vi "Update post-assembly comments.vi"(8 "error in (no error)":errorcluster, 10 "Tray N Pos M":T1, 11 "Stack in":refnum<class "Stack.lvclass">) -> (0 "error out":errorcluster, 3 "Stack out":refnum<class "Stack.lvclass">)   [LabVIEW 2021, in "Stack.lvclass"]
uses:
  Stack.lvclass
  Stack.lvclass/Stack.ctl
panel:
  # "This is only to be used if all data is being written at the same time. If not, skip this vi."
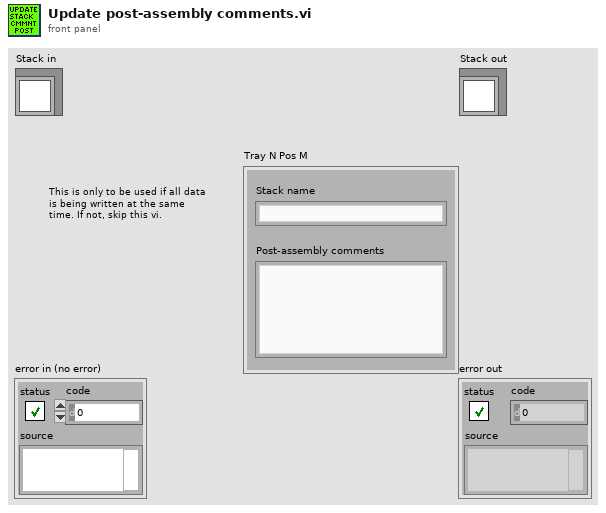
[diagram p1: front panel]
types:
  T1 = cluster{"Stack name":string, "Post-assembly comments":string}
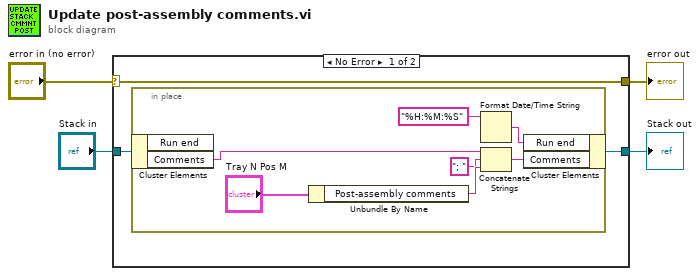
[diagram p0: block diagram]
diagram:
  n1 = case shown="No Error" "error in (no error)" {
    selector: "error in (no error)" -> [w7 w16]
    tunnel: [w7 w16] -> w3
    tunnel: [w5 w15] -> w1
    tunnel: "Stack in" -> [w6 w15]
    frame No Error {
      n2 = in-place {
        n3 = in-place-cluster #1(w6) -> ("Comments"=w11:string)  [unwired: 1 out]
        n4 = Unbundle By Name("Tray N Pos M") -> ("Post-assembly comments"=w10:string)
        n5 = Format Date/Time String(time format string (%c)="%H:%M:%S") -> (date/time string=w13:string)  [unwired: 2 in]
        n6 = Concatenate Strings(w11, "; " ("string"), w10) -> (w9:string)
        n7 = in-place-cluster #1("Run end"=w13, "Comments"=w9) -> (w5:refnum<class "Stack.lvclass">)
      }
    }
    frame Error {
    }
  }
  "error out" <- w3
  "Stack out" <- w1
